vi "InitialMissionImage.vi"() -> ()   [LabVIEW 2011]
panel:
  out "Initial Mission Image":picture
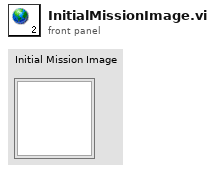
[diagram p1: front panel]
diagram:
